vi "TCP_READ_WAVEFORM.vi"(0 "connection ID":refnum<k5>, 1 "error in (no error)":errorcluster) -> (2 "waveform":waveform(dbl), 3 "connection ID out":refnum<k5>, 4 "error out":errorcluster)   [LabVIEW 2023]
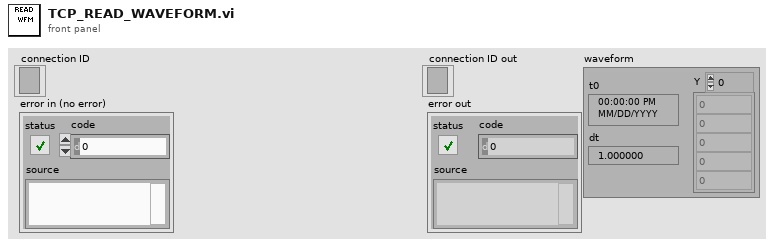
[diagram p1: front panel]
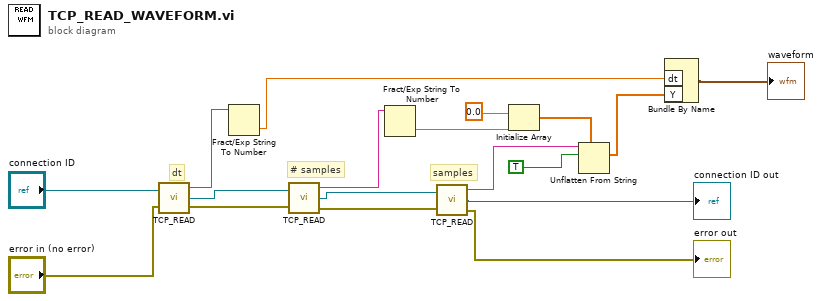
[diagram p0: block diagram]
diagram:
  # "samples"
  # "# samples"
  # "dt"
  n1 = call "TCP_READ.vi"("connection ID"="connection ID", "error in (no error)"="error in (no error)") -> ("data"=w16:string, "connection ID out"=w15:refnum<k5>, "error out"=w14:errorcluster)
  n2 = Fract/Exp String To Number(string=w16) -> (number=w3:dbl)  [unwired: 3 in, 1 out]
  n3 = call "TCP_READ.vi"("connection ID"=w15, "error in (no error)"=w14) -> ("data"=w13:string, "connection ID out"=w12:refnum<k5>, "error out"=w11:errorcluster)
  n4 = Fract/Exp String To Number(string=w13) -> (number=w8:dbl)  [unwired: 3 in, 1 out]
  n5 = call "TCP_READ.vi"("connection ID"=w12, "error in (no error)"=w11) -> ("data"=w5:string, "connection ID out"=→"connection ID out":refnum<k5>, "error out"=→"error out":errorcluster)
  n6 = Initialize Array(0.0 ("element"), w8) -> (w6:dbl[])
  n7 = Unflatten From String(type=w6, binary string=w5, data includes array or string size? (T)=TRUE) -> (value=w2:dbl[])  [unwired: 2 in, 2 out]
  n8 = Bundle By Name("dt"=w3, "Y"=w2) -> (→"waveform":waveform(dbl))  [unwired: 1 in]
